vi "Get Data String.vi"(8 "error in":errorcluster, 11 "IMessage in":refnum<class "IMessage.lvclass">) -> (0 "error out":errorcluster, 2 "Data String":string, 3 "IMessage out":refnum<class "IMessage.lvclass">)   [LabVIEW 2025, in "IMessage.lvclass"]
uses:
  IMessage.lvclass
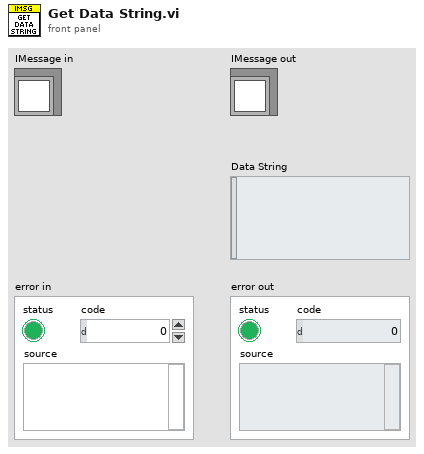
[diagram p1: front panel]
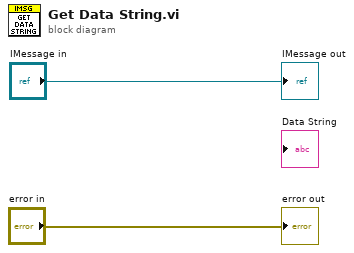
[diagram p0: block diagram]
diagram:
  "IMessage out" <- "IMessage in"
  "error out" <- "error in"
